vi "NXT-HID-Remote.vi"(2 "Transmit Mode":u8(ring)=1 items=["Direct Keyboard data", "Ascii Text data"], 12 "Key Modifier":u8(ring) items=["None"=0, "Left Control Key"=1, "Left Shift Key"=2, "Left Alt Key"=4, "Left GUI Key"=8, "Right Control Key"=16, "Right Shift Key"=32, "Right Alt Key"=64, "Right GUI Key"=128], 13 "Keydata":u8=58 caption="keydata" format="%x", 14 "Text Data":string="NXTHID is writing this ....") -> ()   [LabVIEW 2009]
doc: "Transmission Mode\n0 - Direct Keyboard Data\n1 - Ascii Text Data\n\nPort- Sensor Port NXT-HID is connected to\n\nDevice Adress -Specify the adress of the NXT-HID (Default x04)\n\nIf using Direct Keyboard Data specify the Key Data and Key Modifier if needed.\n\nIf using Ascii Text Data specify the ascii string to send in Text Data"
uses:
  <vilib>/NXT/Block Support/NXT_InputPort.ctl
  <vilib>/NXT/Subs/LVHSConnector.ctl
panel:
  out "Status (boolean)":bool
  out "NXT dup":T1={"error"={"status"=FALSE, "code"=0, "source"=""}, "address"="", "NXT #"=-1, "Show Error"=TRUE}
  in  "NXT":T1={"error"={"status"=FALSE, "code"=0, "source"=""}, "address"="", "NXT #"=-1, "Show Error"=TRUE}
  in  "Input Port":T2 items=["Port 1", "Port 2", "Port 3", "Port 4"]
  # "mindsensors.com\nCopyright (c) 2009 by mindsensors.com\nEmail: info (<at>) mindsensors (<dot>) com\n\nThis program is free software. You can redistribute it and/or modify\nit under the terms of the GNU General Public License as published by\nthe Free Software Foundation; version 3 of the License.\nRead the license at: http://www.gnu.org/licenses/gpl.txt"
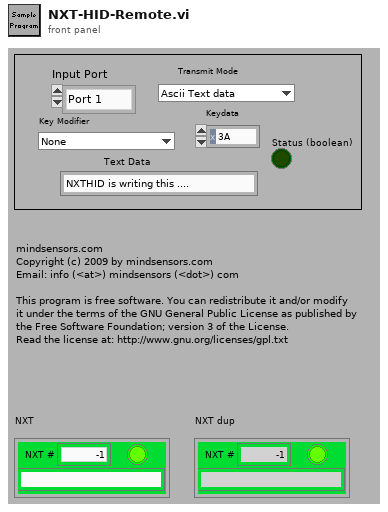
[diagram p1: front panel]
types:
  T1 = typedef "LVHSConnector.ctl" = cluster{"error":errorcluster, "address":string, "NXT #":i32, "Show Error":bool}
  T2 = typedef "NXT_InputPort.ctl" = u8
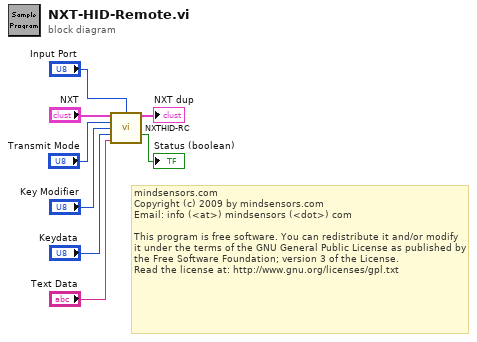
[diagram p0: block diagram]
diagram:
  # "mindsensors.com\nCopyright (c) 2009 by mindsensors.com\nEmail: info (<at>) mindsensors (<dot>) com\n\nThis program is free software. You can redistribute it and/or modify\nit under the terms of the GNU General Public License as published by\nthe Free Software Foundation; version 3 of the License.\nRead the license at: http://www.gnu.org/licenses/gpl.txt"
  n1 = call "NXTHID-RC.vi"("NXT"="NXT", "Input Port"="Input Port", "Transmit Mode"="Transmit Mode", "Key Modifier"="Key Modifier", "Keydata"="Keydata", "Text Data"="Text Data") -> ("NXT dup"=→"NXT dup":T1, "Status (boolean)"=→"Status (boolean)":bool)  [unwired: 8 in]
